vi "sin test.vi"() -> ()   [LabVIEW 2020]
uses:
  <vilib>/rvi/FXPMathLib/FxpSinAndCos/subVIs/nifxpmath_SinAndCos_SimConfig.ctl
  <vilib>/rvi/FXPMathLib/FxpSinAndCos/simVIs/DllFxpSinAndCosTemp_sub.vi
  <vilib>/rvi/FXPMathLib/FxpSinAndCos/XNode/nifxpmath_SinAndCos.xnode
panel:
  out "cos(x)":fxp<+/-,16,2>
  out "sin(x)":fxp<+/-,16,2>
  in  "x (pi)":fxp<+,18,3>
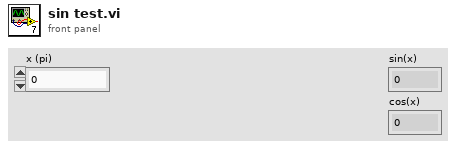
[diagram p1: front panel]
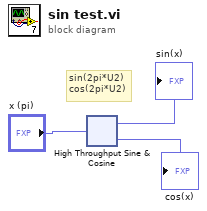
[diagram p0: block diagram]
diagram:
  # "sin(2pi*U2)\ncos(2pi*U2)"
  n1 = xnode "High Throughput Sine & Cosine"("x (pi)"="x (pi)") -> ("sin(x)"=→"sin(x)":fxp<+/-,16,2>, "cos(x)"=→"cos(x)":fxp<+/-,16,2>)
